vi "Do.vi"(8 "error in (no error)":errorcluster, 10 "Actor in":refnum<class "Actor.lvclass">, 11 "MFActorMsg":refnum<class "MFActorMsg.lvclass">) -> (0 "error out":errorcluster, 2 "Actor out":refnum<class "Actor.lvclass">)   [LabVIEW 2024, in "MFActor.lvlib" / "MFActorMsg.lvclass"]
doc: "(<B>Filename</B>: Actor Framework.lvlib:Message.lvclass:Do.vi)\n\nDefines what a message does when it is received by an actor. Generally, a message instructs an actor to invoke one of its methods. By default, this method does nothing. A child class must override it to define behavior. Create a child class by using the Actor Framework Message Maker dialog box."
uses:
  MFActorMsg.lvclass
  <vilib>/ActorFramework/Actor/Actor.lvclass
  MFActor/MFActor.lvclass
  C:/Program Files (x86)/National Instruments/LabVIEW 2024/vi.lib/ActorFramework/Actor/Actor.lvclass
  MFActorMsg.lvclass/MFActorMsg.ctl
  DeviceAlias.ctl
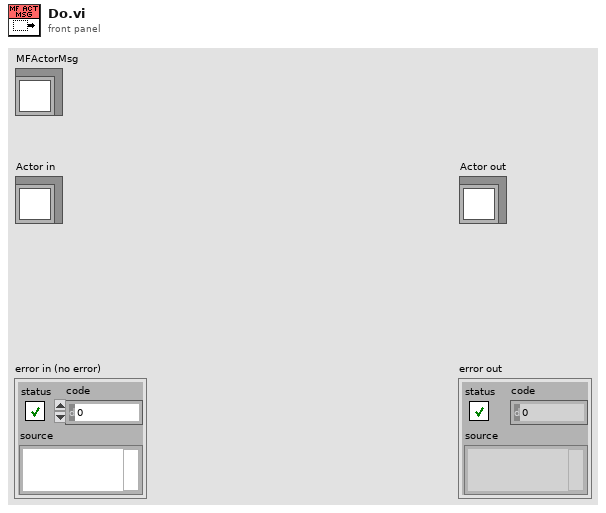
[diagram p1: front panel]
types:
  T1 = typedef "MF Task Name.ctl" = enum16{"DIChanged", "UpdateErrorCode", "SetTorque", "SetDriveTorque", "DataUpdated", "RunningTestProc", "StreamCtrl", "RunPID", "StopTest", "TCP Conn", "RefreshAutoUI", "ZeroAngle"}
  T2 = typedef "DeviceAlias.ctl" = enum16{"TQM0", "TQM1", "PM", "THERMO", "DC POWER"}
  T3 = cluster{bool, "StreamValue":cluster{"Period(sec)":dbl, "WaveCrest":dbl, "WaveTrough":dbl}}
  T4 = cluster{"Period(sec)":dbl, "WaveCrest":dbl, "WaveTrough":dbl}
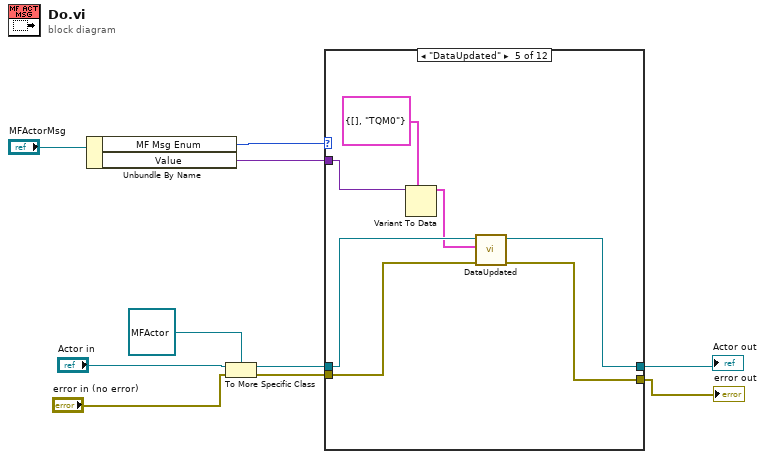
[diagram p0: block diagram]
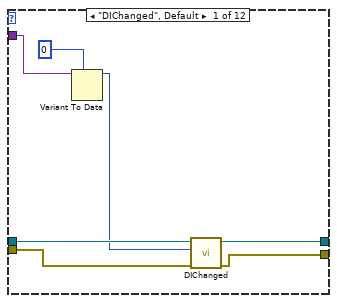
[diagram p2: hidden frame]
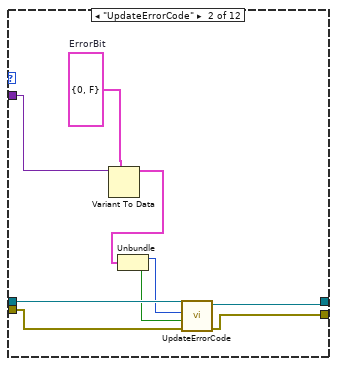
[diagram p3: hidden frame]
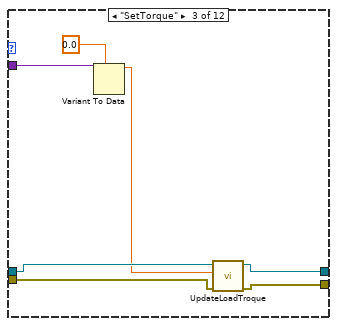
[diagram p4: hidden frame]
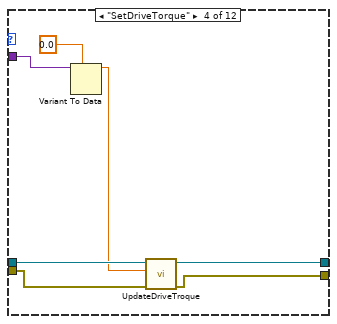
[diagram p5: hidden frame]
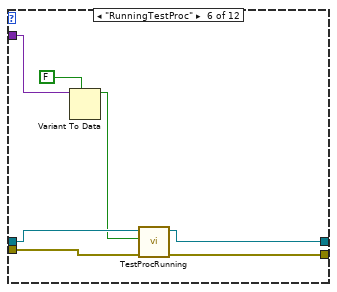
[diagram p6: hidden frame]
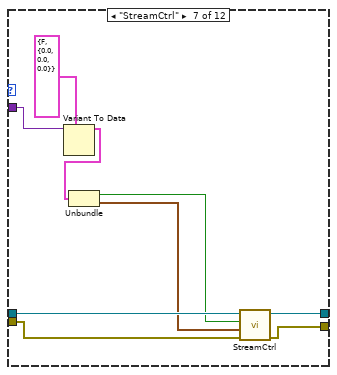
[diagram p7: hidden frame]
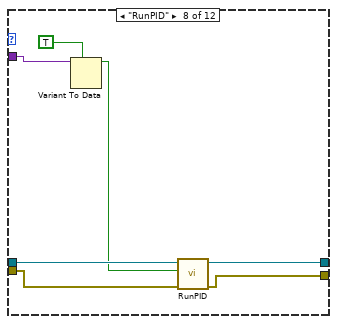
[diagram p8: hidden frame]
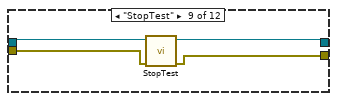
[diagram p9: hidden frame]
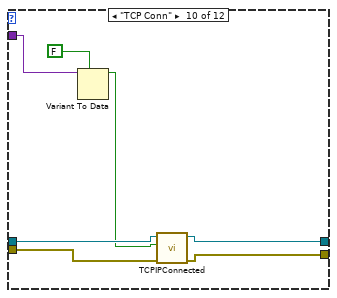
[diagram p10: hidden frame]
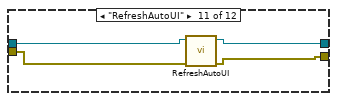
[diagram p11: hidden frame]
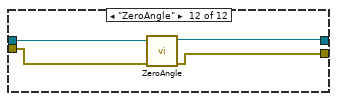
[diagram p12: hidden frame]
diagram:
  n1 = Unbundle By Name("MFActorMsg") -> ("MF Msg Enum"=w9:T1, "Value"=w8:variant)
  n2 = To More Specific Class(target class=refnum<class "MFActor.lvclass"> refnum ("MFActor.lvlib:MFActor.lvclass"), reference="Actor in", error in="error in (no error)") -> (specific class reference=w3:refnum<class "MFActor.lvclass">, error out=w4:errorcluster)
  n3 = case shown="\"DataUpdated\"" w9 {
    tunnel: w8 -> [w13 w21 w33 w38 w43 w50 w63 w70 _ w77 _ _]
    tunnel: w4 -> [w14 w23 w29 w36 w46 w52 w59 w66 w73 w80 w84 w88]
    tunnel: w3 -> [w17 w24 w31 w40 w47 w54 w60 w68 w74 w81 w85 w89]
    tunnel: [w16 w26 w28 w35 w45 w53 w58 w67 w72 w79 w83 w87] -> w2
    tunnel: [w15 w25 w27 w34 w44 w51 w57 w65 w71 w78 w82 w86] -> w1
    frame "DIChanged", Default {
      n4 = Variant To Data(type=u32 0, Variant=w13) -> (data=w11:u32)  [unwired: 1 in, 1 out]
      n5 = call "DIChanged.vi"("error in (no error)"=w14, "DIValue"=w11, "MFActor in"=w17) -> ("error out"=w15:errorcluster, "MFActor out"=w16:refnum<class "MFActor.lvclass">)  [unwired: 7 in]
    }
    frame "UpdateErrorCode" {
      w22 = cluster{"Bit":i32, "Error":bool} {"Bit"=0, "Error"=FALSE}  # ErrorBit
      n6 = Variant To Data(type=w22, Variant=w21) -> (data=w20:cluster{"Bit":i32, "Error":bool})  [unwired: 1 in, 1 out]
      n7 = Unbundle(w20) -> ("Bit"=w19:i32, "Error"=w18:bool)
      n8 = call "UpdateErrorCode.vi"("error in (no error)"=w23, "Error"=w18, "ErrorBit"=w19, "MFActor in"=w24) -> ("error out"=w25:errorcluster, "MFActor out"=w26:refnum<class "MFActor.lvclass">)  [unwired: 6 in]
    }
    frame "SetTorque" {
      n9 = Variant To Data(type=0.0, Variant=w33) -> (data=w30:dbl)  [unwired: 1 in, 1 out]
      n10 = call "UpdateLoadTroque.vi"("error in (no error)"=w29, "TorqueValue(%)"=w30, "MFActor in"=w31) -> ("error out"=w27:errorcluster, "MFActor out"=w28:refnum<class "MFActor.lvclass">)  [unwired: 7 in]
    }
    frame "SetDriveTorque" {
      n11 = Variant To Data(type=0.0, Variant=w38) -> (data=w37:dbl)  [unwired: 1 in, 1 out]
      n12 = call "UpdateDriveTroque.vi"("error in (no error)"=w36, "DriveTQOutput(%)"=w37, "MFActor in"=w40) -> ("error out"=w34:errorcluster, "MFActor out"=w35:refnum<class "MFActor.lvclass">)  [unwired: 7 in]
    }
    frame "DataUpdated" {
      n13 = Variant To Data(type=cluster{dbl[], "Device":T2} {[], "Device"=enum."TQM0"}, Variant=w43) -> (data=w41:cluster{dbl[], "Device":T2})  [unwired: 1 in, 1 out]
      n14 = call "DataUpdated.vi"("error in (no error)"=w46, "TestData"=w41, "MFActor in"=w47) -> ("error out"=w44:errorcluster, "MFActor out"=w45:refnum<class "MFActor.lvclass">)  [unwired: 7 in]
    }
    frame "RunningTestProc" {
      n15 = Variant To Data(type=FALSE, Variant=w50) -> (data=w48:bool)  [unwired: 1 in, 1 out]
      n16 = call "TestProcRunning.vi"("error in (no error)"=w52, "TestProcRunning"=w48, "MFActor in"=w54) -> ("error out"=w51:errorcluster, "MFActor out"=w53:refnum<class "MFActor.lvclass">)  [unwired: 7 in]
    }
    frame "StreamCtrl" {
      n17 = Variant To Data(type=T3 {FALSE, "StreamValue"={"Period(sec)"=0.0, "WaveCrest"=0.0, "WaveTrough"=0.0}}, Variant=w63) -> (data=w61:T3)  [unwired: 1 in, 1 out]
      n18 = Unbundle(w61) -> (w56:bool, "StreamValue"=w55:T4)
      n19 = call "StreamCtrl.vi"("error in (no error)"=w59, "StreamValue"=w55, "Enable"=w56, "MFActor in"=w60) -> ("error out"=w57:errorcluster, "MFActor out"=w58:refnum<class "MFActor.lvclass">)  [unwired: 6 in]
    }
    frame "RunPID" {
      n20 = Variant To Data(type=TRUE, Variant=w70) -> (data=w64:bool)  [unwired: 1 in, 1 out]
      n21 = call "RunPID.vi"("error in (no error)"=w66, "RunPID"=w64, "MFActor in"=w68) -> ("error out"=w65:errorcluster, "MFActor out"=w67:refnum<class "MFActor.lvclass">)  [unwired: 7 in]
    }
    frame "StopTest" {
      n22 = call "StopTest.vi"("error in (no error)"=w73, "MFActor in"=w74) -> ("error out"=w71:errorcluster, "MFActor out"=w72:refnum<class "MFActor.lvclass">)  [unwired: 8 in]
    }
    frame "TCP Conn" {
      n23 = Variant To Data(type=FALSE, Variant=w77) -> (data=w75:bool)  [unwired: 1 in, 1 out]
      n24 = call "TCPIPConnected.vi"("error in (no error)"=w80, "Connected"=w75, "MFActor in"=w81) -> ("error out"=w78:errorcluster, "MFActor out"=w79:refnum<class "MFActor.lvclass">)  [unwired: 7 in]
    }
    frame "RefreshAutoUI" {
      n25 = call "RefreshAutoUI.vi"("error in (no error)"=w84, "MFActor in"=w85) -> ("error out"=w82:errorcluster, "MFActor out"=w83:refnum<class "MFActor.lvclass">)  [unwired: 8 in]
    }
    frame "ZeroAngle" {
      n26 = call "ZeroAngle.vi"("error in (no error)"=w88, "MFActor in"=w89) -> ("error out"=w86:errorcluster, "MFActor out"=w87:refnum<class "MFActor.lvclass">)  [unwired: 8 in]
    }
  }
  "error out" <- w1
  "Actor out" <- w2
